vi "G#Debugger_GetAllClassesInProject.vi"(0 "Active Project":refnum<vi>, 5 "error in (no error)":errorcluster) -> (15 "G#Classes":string[](array[string]), 19 "error out":errorcluster)   [LabVIEW 2017, in "G#Debugger.lvlib"]
uses:
  G#Debugger.lvlib
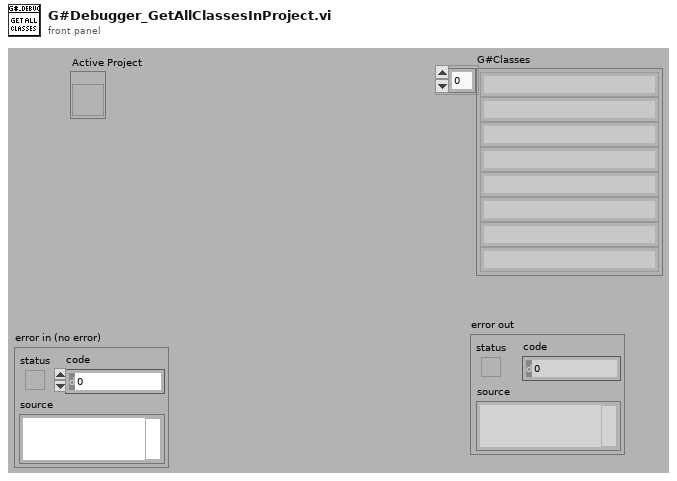
[diagram p1: front panel]
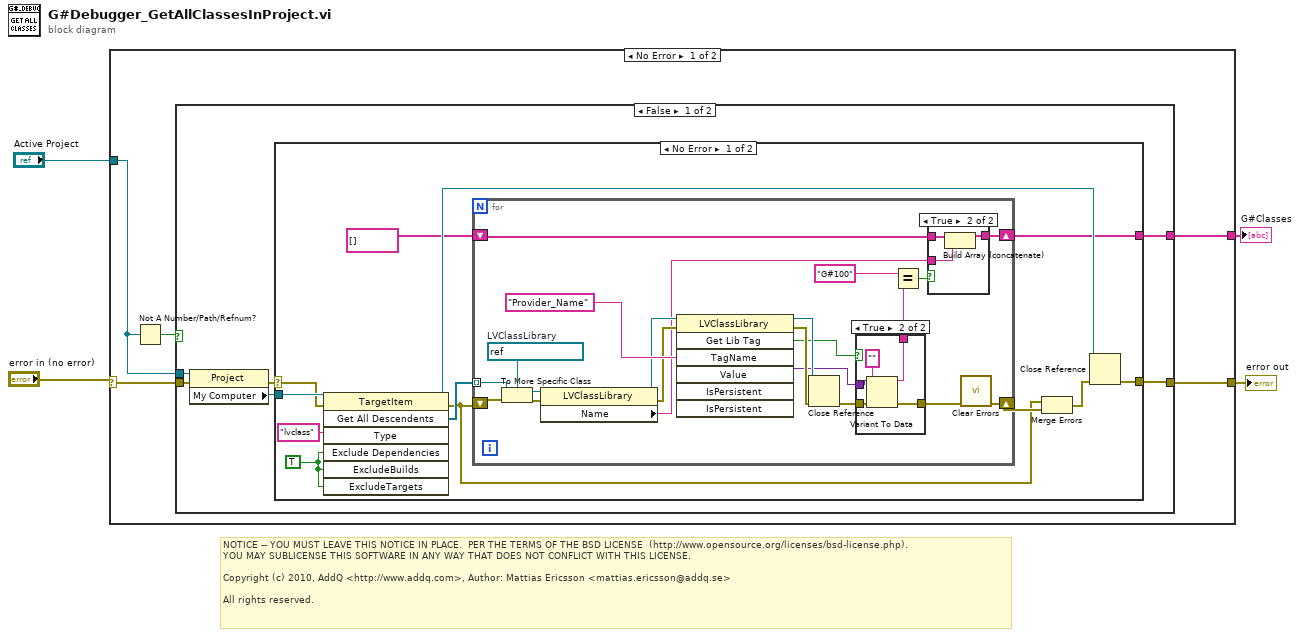
[diagram p0: block diagram]
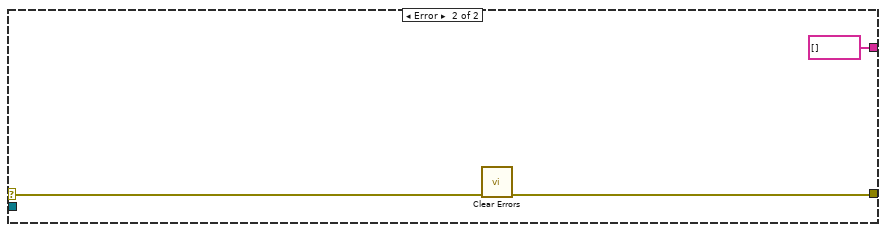
[diagram p4: hidden frame]
diagram:
  # "NOTICE -- YOU MUST LEAVE THIS NOTICE IN PLACE.  PER THE TERMS OF THE BSD LICENSE  (http://www.opensource.org/licenses/bsd-license.php).\nYOU MAY SUBLICENSE THIS SOFTWARE IN ANY WAY THAT DOES NOT CONFLICT WITH THIS LICENSE.\n\nCopyright (c) 2010, AddQ <http://www.addq.com>, Author: Mattias Ericsson <mattias.ericsson@addq.se>\n\nAll rights reserved."
  n1 = case shown="No Error" "error in (no error)" {
    selector: "error in (no error)" -> [w7 w63]
    tunnel: [w5 w63] -> w3
    tunnel: [w9 _] -> w2
    tunnel: "Active Project" -> [w6 _]
    frame No Error {
      n2 = Not A Number/Path/Refnum?(number/path/refnum=w6) -> (NaN/Path/Refnum?=w8:bool)
      n3 = case shown="False" w8 {
        tunnel: w7 -> [w14 w62]
        tunnel: [w11 w62] -> w5
        tunnel: [w13 _] -> w9
        tunnel: w6 -> [w12 _]
        frame False {
          n4 = property class="Project"(reference=w12, error in=w14) -> (error out=w10:errorcluster, "My Computer"=w15:refnum<vi>)  [unwired: 1 out]
          n5 = case shown="No Error" w10 {
            selector: w10 -> [w16 w61]
            tunnel: w15 -> [w27 _]
            tunnel: [w19 string[] [] ("G#Classes")] -> w13
            tunnel: [w18 w60] -> w11
            frame No Error {
              w17 = TRUE ("ExcludeDependencies")
              n6 = invoke class="TargetItem" method="Get All Descendents"(reference=w27, error in=w16, "Type"="lvclass", "Exclude Dependencies"=w17, "ExcludeBuilds"=w17, "ExcludeTargets"=w17) -> (reference out=w21:refnum<vi>, error out=w23:errorcluster, "All Descendents"=w25:refnum<vi>[])  [unwired: 1 in, 4 out]
              n7 = for {
                shift-right: [w40] -> w24
                shift-left: w23 -> [w48]
                tunnel: w25 -> [w47] mode=indexing
                shift-right: [w35] -> w19
                shift-left: string[] [] ("G#Classes") -> [w34]
                w46 = refnum<vi> refnum  # LVClassLibrary
                n8 = To More Specific Class(target class=w46, reference=w47, error in=w48) -> (specific class reference=w31:refnum<vi>, error out=w33:errorcluster)
                n9 = property class="LVClassLibrary"(reference=w31, error in=w33) -> (reference out=w30:refnum<vi>, error out=w32:errorcluster, "Name"=w29:string)
                n10 = invoke class="LVClassLibrary" method="Get Lib Tag"(reference=w30, error in=w32, "TagName"="Provider_Name") -> (reference out=w44:refnum<vi>, error out=w43:errorcluster, "GetTag"=w28:bool, "Value"=w41:variant)  [unwired: 4 in, 3 out]
                n11 = Close Reference(reference=w44, error in (no error)=w43) -> (error out=w42:errorcluster)
                n12 = case shown="True" w28 {
                  tunnel: w42 -> [w49 w54]
                  tunnel: w41 -> [_ w52]
                  tunnel: [w49 w51] -> w39
                  tunnel: [_ w50] -> w38
                  frame False {
                  }
                  frame True {
                    n13 = Variant To Data(error in=w54, type="", Variant=w52) -> (data=w50:string, error out=w51:errorcluster)
                  }
                }
                n14 = Equal?(x="G#100", y=w38) -> (x = y?=w36:bool)
                n15 = case shown="True" w36 {
                  tunnel: [w55 w58] -> w35
                  tunnel: w34 -> [w55 w57]
                  tunnel: w29 -> [_ w56]
                  frame False {
                  }
                  frame True {
                    n16 = Build Array (concatenate)(w57, w56) -> (w58:string[])
                  }
                }
                n17 = call <vilib>:"Clear Errors.vi"("error in (no error)"=w39) -> ("error out"=w40:errorcluster)  [unwired: 5 in, 1 out]
              }
              n18 = Merge Errors(w23, w24) -> (w22:errorcluster)
              n19 = Close Reference(reference=w21, error in (no error)=w22) -> (error out=w18:errorcluster)
            }
            frame Error {
              n20 = call <vilib>:"Clear Errors.vi"("error in (no error)"=w61) -> ("error out"=w60:errorcluster)  [unwired: 5 in, 1 out]
            }
          }
        }
        frame True {
        }
      }
    }
    frame Error {
    }
  }
  "error out" <- w3
  "G#Classes" <- w2
